vi "LWXPS_PositionerExcitationSignalGet.vi"(0 "XPS Reference IN":refnum<k24>, 2 "Positioner Name":string, 5 "LabVIEW error IN":errorcluster) -> (12 "XPS Reference OUT":refnum<k24>, 13 "LabVIEW error OUT":errorcluster, 14 "Returned error code":i32, 15 "Mode":i32, 16 "Frequency":dbl, 17 "Amplitude":dbl, 18 "Time":dbl, 19 "XPS Error String":string)   [LabVIEW 2014]
uses:
  D:/XPSQ8_LabView_Library/Development/Source/Dll/Newport.XPS.CommandInterface.dll
  Dll/Newport.XPS.CommandInterface.dll
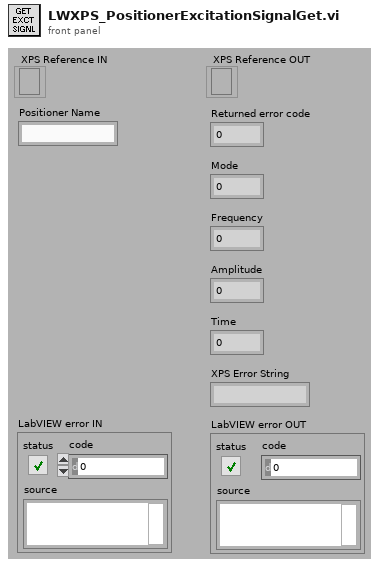
[diagram p1: front panel]
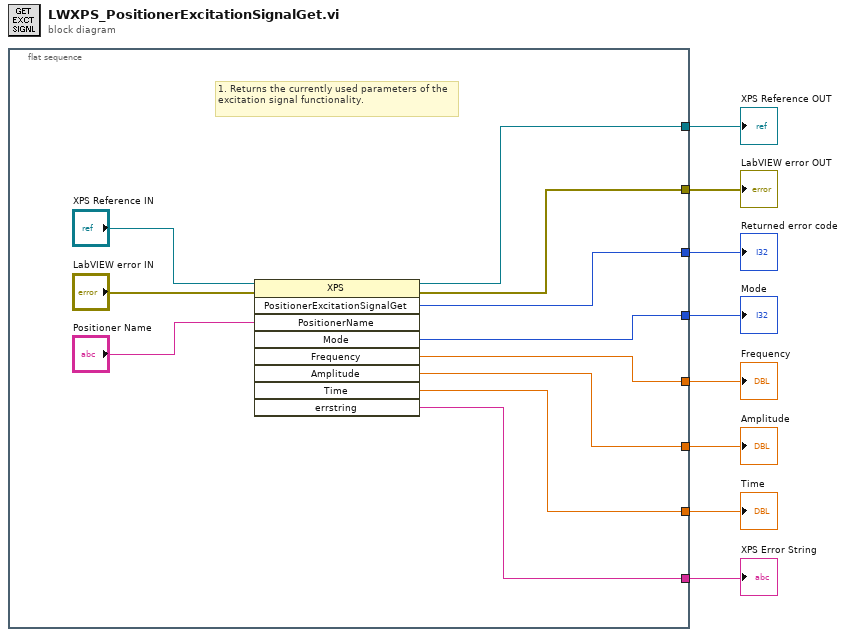
[diagram p0: block diagram]
diagram:
  n1 = flat-sequence {
    tunnel: [w17] -> w8
    tunnel: [w15] -> w7
    tunnel: [w18] -> w6
    tunnel: [w10] -> w1
    tunnel: [w14] -> w5
    tunnel: [w13] -> w4
    tunnel: [w12] -> w2
    tunnel: [w11] -> w3
    frame #0 {
      # "1. Returns the currently used parameters of the excitation signal functionality."
      n2 = invoke class="XPS" method="PositionerExcitationSignalGet"(reference="XPS Reference IN", error in="LabVIEW error IN", "PositionerName"="Positioner Name") -> (reference out=w17:refnum<k24>, error out=w15:errorcluster, "PositionerExcitationSignalGet"=w18:i32, "Mode"=w10:i32, "Frequency"=w14:dbl, "Amplitude"=w13:dbl, "Time"=w12:dbl, "errstring"=w11:string)  [unwired: 6 in, 1 out]
    }
  }
  "XPS Error String" <- w3
  "XPS Reference OUT" <- w8
  "LabVIEW error OUT" <- w7
  "Returned error code" <- w6
  "Frequency" <- w5
  "Amplitude" <- w4
  "Time" <- w2
  "Mode" <- w1
